vi "client_chat2.vi"() -> ()   [LabVIEW 2024]
panel:
  in  "stop":bool
  out "String":string
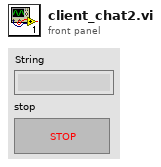
[diagram p1: front panel]
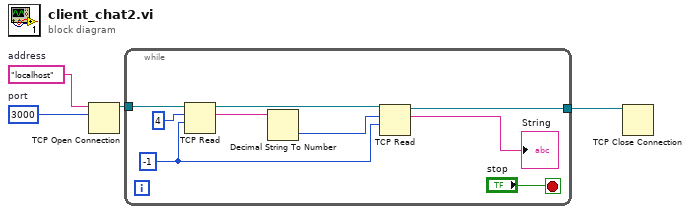
[diagram p0: block diagram]
diagram:
  w3 = u16 3000  # port
  w4 = "localhost"  # address
  n1 = TCP Open Connection(address=w4, remote port or service name=w3) -> (connection ID=w2:refnum<k5>)  [unwired: 1 in, 3 out]
  n2 = while {
    tunnel: w2 -> [w9]
    tunnel: [w13] -> w1
    stop <- "stop" stop-if-true
    w10 = -1 ("timeout ms (25000)")
    n3 = TCP Read(connection ID=w9, bytes to read=4, 9:w10) -> (connection ID out=w7:refnum<k5>, data out=w6:string)  [unwired: 1 in, 2 out]
    n4 = Decimal String To Number(string=w6) -> (number=w5:i32)  [unwired: 2 in, 1 out]
    n5 = TCP Read(connection ID=w7, bytes to read=w5, 9:w10) -> (connection ID out=w13:refnum<k5>, data out=→"String":string)  [unwired: 1 in, 2 out]
  }
  n6 = TCP Close Connection(connection ID=w1) -> ()  [unwired: 1 in, 3 out]
